vi "Build Private Data.vi"(8 "error in (no error)":errorcluster, 9 "Wiring Spec":T1, 11 "CS++Actor in":refnum<class "CS++Actor.lvclass">) -> (0 "error out":errorcluster, 3 "CS++Actor out":refnum<class "CS++Actor.lvclass">)   [LabVIEW 2014, in "CS++Actor.lvlib" / "CS++Actor.lvclass"]
doc: "creates the attribute data of the new message."
uses:
  CS++Actor.lvclass
  <vilib>/Utility/traverseref.llb/TRef TravTarget.ctl
  CS++Actor.lvclass/CS++Actor.ctl
  <vilib>/Utility/miscctls.llb/LVPositionTypeDef.ctl
  <vilib>/Utility/traverseref.llb/VI Scripting - Traverse.lvlib
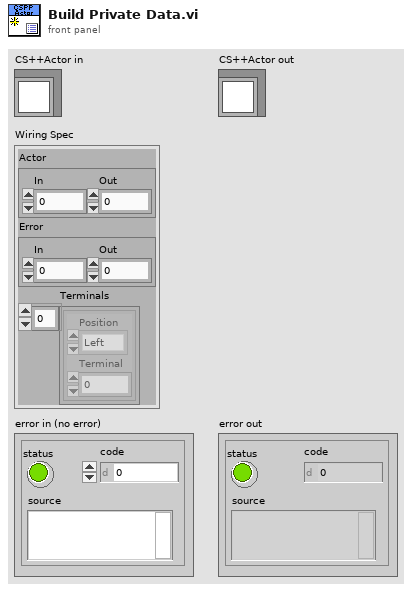
[diagram p1: front panel]
types:
  T1 = cluster{"Actor":cluster{"In":i32, "Out":i32}, "Error":cluster{"In":i32, "Out":i32}, "Terminals":cluster{"Position":enum16{"Left", "Top", "Bottom", "Right"}, "Terminal":i32}[]}
  T2 = typedef "TRef TravTarget.ctl" = enum16{"FP", "BD", "Other"}
  T3 = typedef "LVPositionTypeDef.ctl" = cluster{"Left":i32, "Top":i32}
  T4 = cluster{"Position":enum16{"Left", "Top", "Bottom", "Right"}, "Terminal":i32}[]
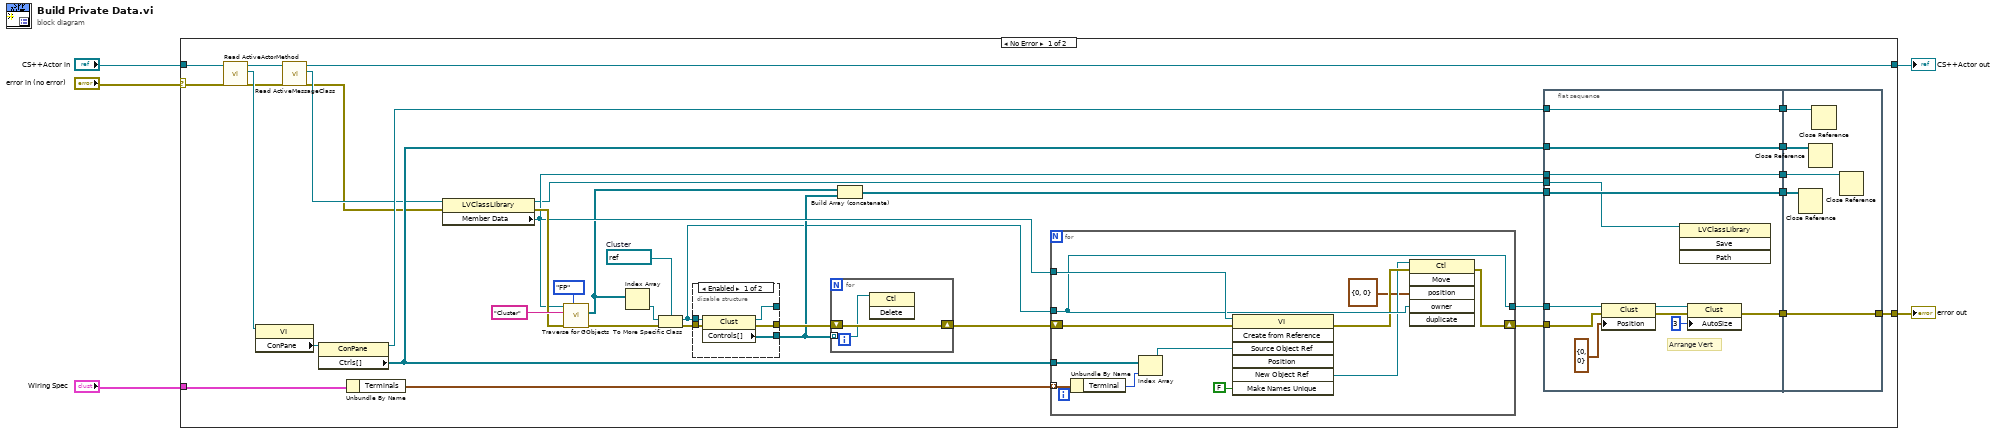
[diagram p0: block diagram]
diagram:
  n1 = case shown="No Error" "error in (no error)" {
    selector: "error in (no error)" -> [w6 w81]
    tunnel: [w27 w81] -> w5
    tunnel: "Wiring Spec" -> [w25 _]
    tunnel: "CS++Actor in" -> [w12 w80]
    tunnel: [w9 w80] -> w2
    frame No Error {
      w31 = refnum<vi> refnum  # Cluster
      n2 = call "Read ActiveActorMethod.vi"("error in (no error)"=w6, "CS++Actor in"=w12) -> ("error out"=w8:errorcluster, "ActiveActorMethod"=w10:refnum<vi>, "CS++Actor out"=w11:refnum<class "CS++Actor.lvclass">)  [unwired: 7 in]
      n3 = property class="VI"(reference=w10) -> ("ConPane"=w36:refnum<vi>)  [unwired: 1 in, 2 out]
      n4 = call "Read ActiveMessageClass.vi"("error in (no error)"=w8, "CS++Actor in"=w11) -> ("error out"=w7:errorcluster, "ActiveMessageClass"=w13:refnum<vi>, "CS++Actor out"=w9:refnum<class "CS++Actor.lvclass">)  [unwired: 7 in]
      n5 = property class="ConPane"(reference=w36) -> (reference out=w16:refnum<vi>, "Ctrls[]"=w26:refnum<vi>[])  [unwired: 1 in, 1 out]
      n6 = Unbundle By Name(w25) -> ("Terminals"=w24:T4)
      n7 = property class="LVClassLibrary"(reference=w13, error in=w7) -> (reference out=w15:refnum<vi>, error out=w33:errorcluster, "Member Data"=w29:refnum<vi>)
      n8 = call <vilib>:"Traverse for GObjects.vi"("Traverse Target"=TRef_TravTarget."FP", "error in (no error)"=w33, "Class Name"="Cluster" ("name/order"), "VI Refnum"=w29) -> ("error out"=w30:errorcluster, "References"=w28:refnum<vi>[])  [unwired: 4 in, 2 out]
      n9 = Index Array(array=w28) -> (element=w32:refnum<vi>)  [unwired: 1 in]
      n10 = To More Specific Class(target class=w31, reference=w32, error in=w30) -> (specific class reference=w14:refnum<vi>, error out=w23:errorcluster)
      n11 = disable-structure shown="Enabled" {
        disable-tunnel: w14 -> [w48 w50]
        disable-tunnel: w23 -> [w47 w49]
        disable-tunnel: [w46 w50] -> _
        disable-tunnel: [w45 w49] -> w20
        disable-tunnel: [w44 _] -> w17
        frame Enabled {
          n12 = property class="Clust"(reference=w48, error in=w47) -> (reference out=w46:refnum<vi>, error out=w45:errorcluster, "Controls[]"=w44:refnum<vi>[])
        }
        frame Disabled {
        }
      }
      n13 = for {
        shift-right: [w43] -> w19
        shift-left: w20 -> [w43]
        tunnel: w17 -> [w42] mode=indexing
        n14 = invoke class="Ctl" method="Delete"(reference=w42) -> ()  [unwired: 2 in, 3 out]
      }
      n15 = Build Array (concatenate)(w28, w17) -> (w18:refnum<vi>[])
      n16 = for {
        tunnel: w26 -> [w75]
        tunnel: w29 -> [w79]
        shift-right: [w78] -> w21
        shift-left: w19 -> [w73]
        tunnel: w24 -> [w74] mode=indexing
        tunnel: w14 -> [w77]
        tunnel: [w77] -> w22
        n17 = Unbundle By Name(w74) -> ("Terminal"=w72:i32)
        n18 = Index Array(array=w75, index=w72) -> (element=w71:refnum<vi>)
        n19 = invoke class="VI" method="Create from Reference"(reference=w79, error in=w73, "Source Object Ref"=w71, "Make Names Unique"=FALSE ("Make Names Unique (F)")) -> (error out=w76:errorcluster, "New Object Ref"=w70:refnum<vi>)  [unwired: 3 in, 5 out]
        n20 = invoke class="Ctl" method="Move"(reference=w70, error in=w76, "position"=T3 {"Left"=0, "Top"=0}, "owner"=w77) -> (error out=w78:errorcluster)  [unwired: 2 in, 5 out]
      }
      n21 = flat-sequence {
        tunnel: w22 -> [w62]
        tunnel: w21 -> [w57]
        tunnel: w29 -> [w54]
        tunnel: w18 -> [w56]
        tunnel: [w53] -> w41
        tunnel: [w54] -> w40
        tunnel: [w56] -> w39
        tunnel: w26 -> [w55]
        tunnel: [w55] -> w38
        tunnel: w16 -> [w52]
        tunnel: [w52] -> w37
        tunnel: w15 -> [w51]
        tunnel: [w67] -> w27
        tunnel: w41 -> [w67]
        tunnel: w40 -> [w66]
        tunnel: w39 -> [w65]
        tunnel: w38 -> [w64]
        tunnel: w37 -> [w63]
        frame #0 {
          # "Arrange Vert"
          n22 = property class="Clust"(reference=w62, error in=w57, "Position"=T3 {"Left"=0, "Top"=0}) -> (reference out=w60:refnum<vi>, error out=w59:errorcluster)
          n23 = invoke class="LVClassLibrary" method="Save"(reference=w51) -> ()  [unwired: 3 in, 4 out]
          n24 = property class="Clust"(reference=w60, error in=w59, "AutoSize"=u32 3 ("Auto Sizing")) -> (error out=w53:errorcluster)  [unwired: 1 out]
        }
        frame #1 {
          n25 = Close Reference(reference=w65) -> ()  [unwired: 1 in, 1 out]
          n26 = Close Reference(reference=w64) -> ()  [unwired: 1 in, 1 out]
          n27 = Close Reference(reference=w63) -> ()  [unwired: 1 in, 1 out]
          n28 = Close Reference(reference=w66) -> ()  [unwired: 1 in, 1 out]
        }
      }
    }
    frame Error {
    }
  }
  "error out" <- w5
  "CS++Actor out" <- w2
